vi "Run_Core.vi"(0 "Message Popup in":refnum<class "UI Functions.lvclass">, 11 "error in (no error)":errorcluster) -> (4 "Message Popup out":refnum<class "UI Functions.lvclass">, 6 "Return":variant, 15 "error out":errorcluster)   [LabVIEW 2019, in "UI Functions.lvclass"]
uses:
  UI Functions.lvclass
  D:/Pet Projects/LSL/source code/LSL components/functions/functionsbase/functionbase.lvclass
  UI Functions.lvclass/UI Functions.ctl
  functionsbase/functionbase.lvclass/functionbase.ctl
  functionsbase/properties/Read Output Terminal.vi
  output terminal/Base/Output Terminal.lvclass
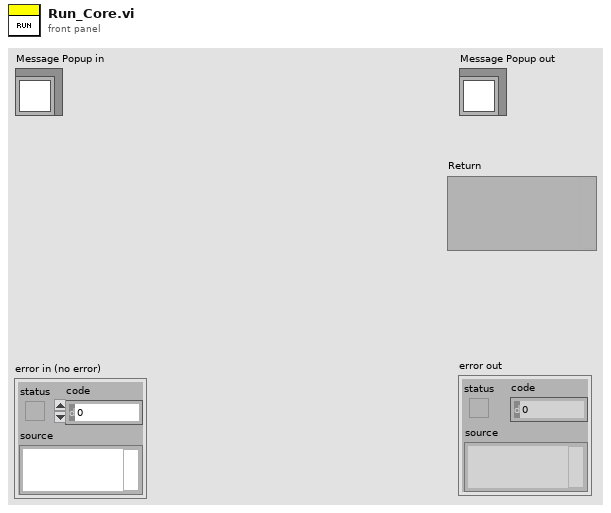
[diagram p1: front panel]
types:
  T1 = typedef "UI Functions.lvclass/Function List.ctl" = enum16{"popup", "print", "Get Bool", "Get Number", "Get String"}
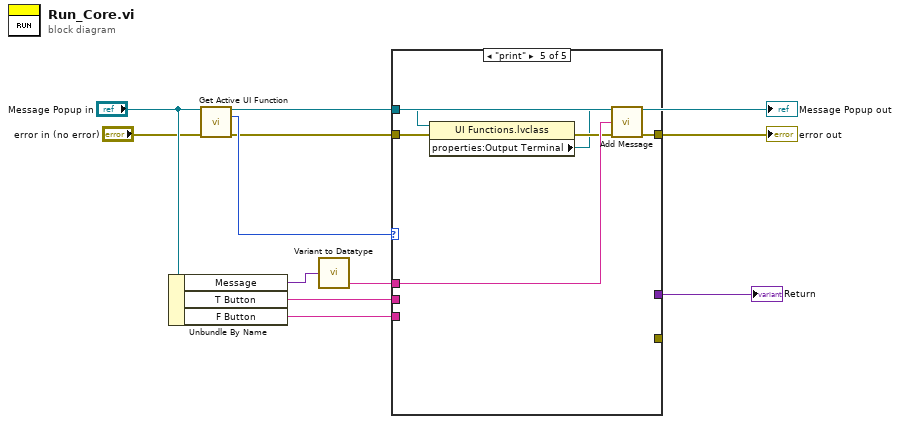
[diagram p0: block diagram]
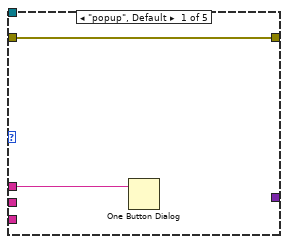
[diagram p2: hidden frame]
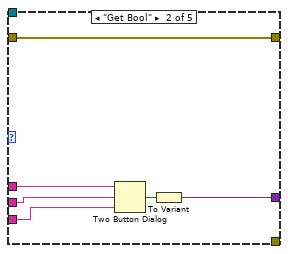
[diagram p3: hidden frame]
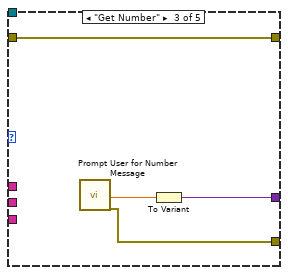
[diagram p4: hidden frame]
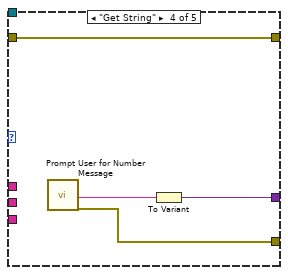
[diagram p5: hidden frame]
diagram:
  n1 = Unbundle By Name("Message Popup in") -> ("Message"=w8:variant, "T Button"=w11:string, "F Button"=w10:string)
  n2 = call "Get Active UI Function.vi"("UI Functions in"="Message Popup in", "error in (no error)"="error in (no error)") -> ("UI Functions out"=w2:refnum<class "UI Functions.lvclass">, "Function List"=w4:T1, "error out"=w3:errorcluster)  [unwired: 11 in]
  "Message Popup out" <- w2
  n3 = call "Variant to Datatype.vi"("Variant"=w8) -> ("Value"=w7:string)  [unwired: 2 in, 2 out]
  n4 = case shown="\"print\"" w4 {
    tunnel: w7 -> [w13 w19 _ _ w33]
    tunnel: w11 -> [_ w18 _ _ _]
    tunnel: w10 -> [_ w17 _ _ _]
    tunnel: [_ w15 w23 w27 _] -> w9
    tunnel: [_ _ w22 w26 _] -> _
    tunnel: w3 -> [w12 w14 w20 w24 w32]
    tunnel: w2 -> [_ _ _ _ w30]
    tunnel: [w12 w14 w20 w24 w28] -> w1
    frame "popup", Default {
      n5 = One Button Dialog(message=w13) -> ()  [unwired: 1 in, 1 out]
    }
    frame "Get Bool" {
      n6 = Two Button Dialog(message=w19, 1:w17, 2:w18) -> (T button?=w16:bool)
      n7 = To Variant(anything=w16) -> (Variant=w15:variant)
    }
    frame "Get Number" {
      n8 = call "Prompt User for Number Message"() -> ("Number"=w21:dbl, "error out"=w22:errorcluster)  [unwired: 17 in, 1 out]
      n9 = To Variant(anything=w21) -> (Variant=w23:variant)
    }
    frame "Get String" {
      n10 = call "Prompt User for Number Message"() -> ("String"=w25:string, "error out"=w26:errorcluster)  [unwired: 17 in, 1 out]
      n11 = To Variant(anything=w25) -> (Variant=w27:variant)
    }
    frame "print" {
      n12 = property class="UI Functions.lvclass"(reference=w30, error in=w32) -> (error out=w31:errorcluster, "properties:Output Terminal"=w29:refnum<class "Output Terminal.lvclass">)  [unwired: 1 out]
      n13 = call-dynamic "Add Message.vi"("Output Terminal in"=w29, "Message"=w33, "error in (no error)"=w31) -> ("error out"=w28:errorcluster)  [unwired: 11 in, 1 out]
    }
  }
  "error out" <- w1
  "Return" <- w9
